vi "Initialize Settings.vi"(8 "error in (no error)":errorcluster, 10 "settings":T1, 11 "GE Reflective Memory Transceiver in":refnum<class "GE Reflective Memory Transceiver.lvclass">) -> (0 "error out":errorcluster, 3 "GE Reflective Memory Transceiver out":refnum<class "GE Reflective Memory Transceiver.lvclass">)   [LabVIEW 2017, in "GE Reflective Memory.lvlib" / "GE Reflective Memory Transceiver.lvclass"]
uses:
  GE Reflective Memory Transceiver.lvclass
  Builds/Data Sharing Framework/Current/Core/DSF Core.lvlibp/Typedefs/DSF Settings Info.ctl
  GE Reflective Memory Transceiver.lvclass/GE Reflective Memory Transceiver.ctl
  <vilib>/NI/GE Reflective Memory Driver/Typedefs/GE 5565PIORC.Typedef.DMA Wait Mode.ctl
  <vilib>/NI/GE Reflective Memory Driver/GE 5565PIORC.lvclass
  Builds/Data Sharing Framework/Current/Core/DSF Core.lvlibp/Classes/Configuration/Configuration Session.lvclass
  Builds/Data Sharing Framework/Current/Core/DSF Core.lvlibp
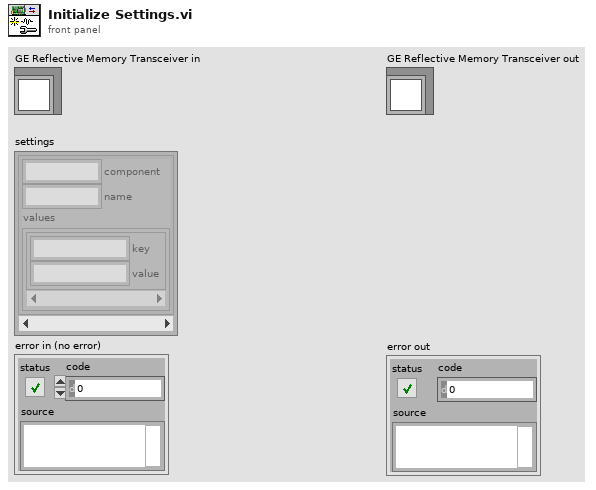
[diagram p1: front panel]
types:
  T1 = typedef "DSF Core.lvlibp/DSF Settings Info.ctl" = cluster{"component":string, "name":string, "values":cluster{"key":string, "value":string}[]}[]
  T2 = typedef "GE 5565PIORC.lvclass/GE 5565PIORC.Typedef.DMA Wait Mode.ctl" = enum16{"Interrupt", "Polling"}
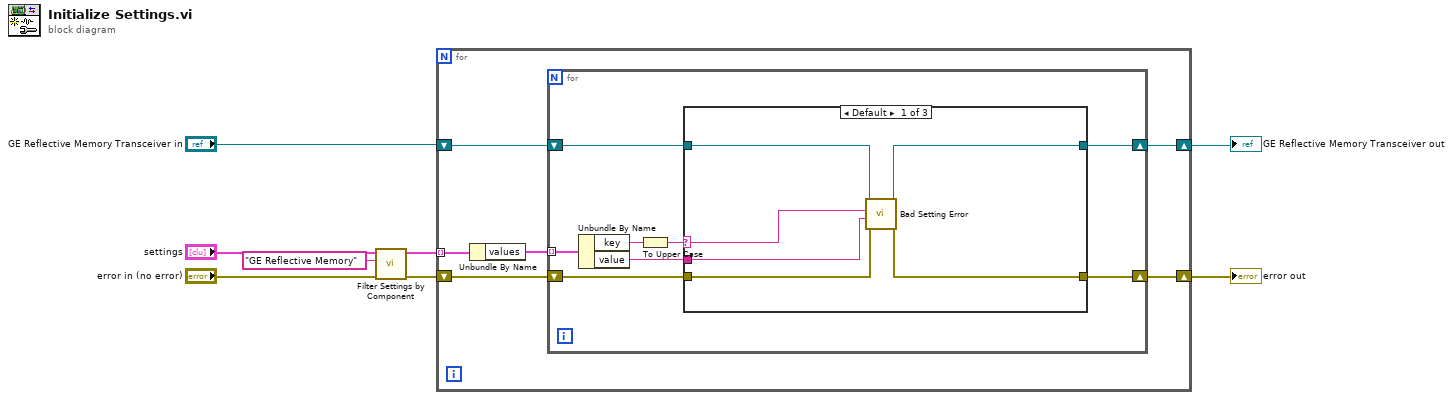
[diagram p0: block diagram]
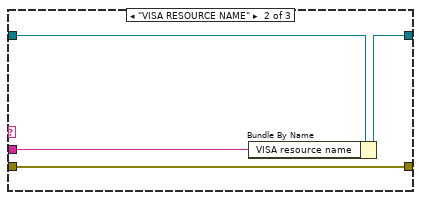
[diagram p2: hidden frame]
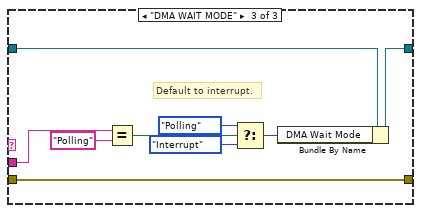
[diagram p3: hidden frame]
diagram:
  n1 = call "Filter Settings by Component.vi"("error in (no error)"="error in (no error)", "component"="GE Reflective Memory", "settings"="settings") -> ("error out"=w1:errorcluster, "filtered settings"=w4:T1)  [unwired: 7 in]
  n2 = for {
    tunnel: w4 -> [w14] mode=indexing
    shift-right: [w12] -> w7
    shift-left: "GE Reflective Memory Transceiver in" -> [w13]
    shift-right: [w10] -> w8
    shift-left: w1 -> [w11]
    n3 = Unbundle By Name(w14) -> ("values"=w9:cluster{"key":string, "value":string}[])
    n4 = for {
      shift-right: [w21] -> w12
      shift-left: w13 -> [w22]
      shift-right: [w19] -> w10
      shift-left: w11 -> [w20]
      tunnel: w9 -> [w18] mode=indexing
      n5 = Unbundle By Name(w18) -> ("key"=w17:string, "value"=w16:string)
      n6 = To Upper Case(1:w17) -> (0:w15:string)
      n7 = case shown="Default" w15 {
        selector: w15 -> [w24 _ _]
        tunnel: w16 -> [w23 w29 w38]
        tunnel: w22 -> [w26 w32 w41]
        tunnel: [w25 w31 w40] -> w21
        tunnel: w20 -> [w28 w30 w39]
        tunnel: [w27 w30 w39] -> w19
        frame Default {
          n8 = call "Bad Setting Error.vi"("error in (no error)"=w28, "value"=w23, "key"=w24, "GE Reflective Memory Transceiver in"=w26) -> ("error out"=w27:errorcluster, "GE Reflective Memory Transceiver out"=w25:refnum<class "GE Reflective Memory Transceiver.lvclass">)  [unwired: 6 in]
        }
        frame "VISA RESOURCE NAME" {
          n9 = Bundle By Name(cluster=w32, "VISA resource name"=w29) -> (w31:refnum<class "GE Reflective Memory Transceiver.lvclass">)
        }
        frame "DMA WAIT MODE" {
          # "Default to interrupt."
          n10 = Equal?(x=w38, y="Polling") -> (x = y?=w36:bool)
          n11 = Select(t=GE_5565PIORC.Typedef.DMA_Wait_Mode."Polling" ("DMA Wait Mode"), s=w36, f=GE_5565PIORC.Typedef.DMA_Wait_Mode."Interrupt" ("DMA Wait Mode")) -> (s? t:f=w35:T2)
          n12 = Bundle By Name(cluster=w41, "DMA Wait Mode"=w35) -> (w40:refnum<class "GE Reflective Memory Transceiver.lvclass">)
        }
      }
    }
  }
  "error out" <- w8
  "GE Reflective Memory Transceiver out" <- w7
